vi "Configure Waveform Modulation Function.vi"(6 "Waveform Rising Time (50)":dbl=50.0, 8 "error in (no error)":errorcluster, 9 "Modulating Signal Shape (0: Sinusoid)":i32(ring) items=["Sinusoid", "Square", "Ramp"], 10 "Waveform Generator Number (1 Waveform Generator 1)":i32(ring)=1 items=["Waveform Generator 1"=1], 11 "VISA resource name":refnum<visa-resource-name>) -> (0 "error out":errorcluster, 3 "VISA resource name out":refnum<visa-resource-name>)   [LabVIEW 2023, in "Keysight-DSQx3014T.lvlib"]
doc: "Specifies the modulating waveform shape and the amount of time per cycle that it is rising."
uses:
  Keysight-DSQx3014T.lvlib
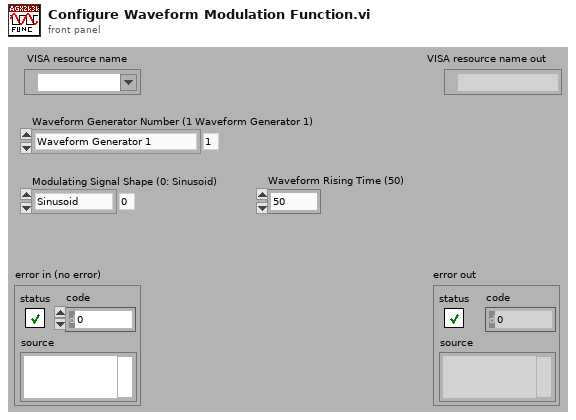
[diagram p1: front panel]
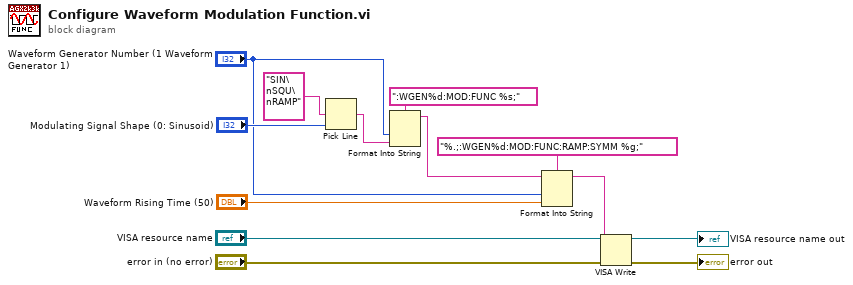
[diagram p0: block diagram]
diagram:
  n1 = Pick Line(multi-line string="SIN\nSQU\nRAMP", line index="Modulating Signal Shape (0: Sinusoid)") -> (output string=w7:string)  [unwired: 1 out]
  n2 = Format Into String(format string=":WGEN%d:MOD:FUNC %s;", "Waveform Generator Number (1 Waveform Generator 1)", w7) -> (resulting string=w6:string)  [unwired: 2 in, 1 out]
  n3 = Format Into String(format string="%.;:WGEN%d:MOD:FUNC:RAMP:SYMM %g;", initial string=w6, "Waveform Generator Number (1 Waveform Generator 1)", "Waveform Rising Time (50)") -> (resulting string=w5:string)  [unwired: 1 in, 1 out]
  n4 = VISA Write(VISA resource name="VISA resource name", write buffer=w5, error in (no error)="error in (no error)") -> (VISA resource name out=→"VISA resource name out":refnum<visa-resource-name>, error out=→"error out":errorcluster)  [unwired: 1 out]
